vi "Read Parameters to process.vi"(8 "error in":errorcluster, 11 "Temperature Controller Logic runtime in":refnum<class "Temperature Controller Logic runtime.lvclass">) -> (0 "error out":errorcluster, 2 "Parameters to process":T1, 3 "Temperature Controller Logic runtime out":refnum<class "Temperature Controller Logic runtime.lvclass">)   [LabVIEW 2015, in "Temperature Controller Logic runtime.lvclass"]
uses:
  Temperature Controller Logic runtime.lvclass
  configuration/parameter data indices.ctl
  Temperature Controller Logic runtime.lvclass/Temperature Controller Logic runtime.ctl
  configuration/Temperature Controller Logic configuration.lvclass
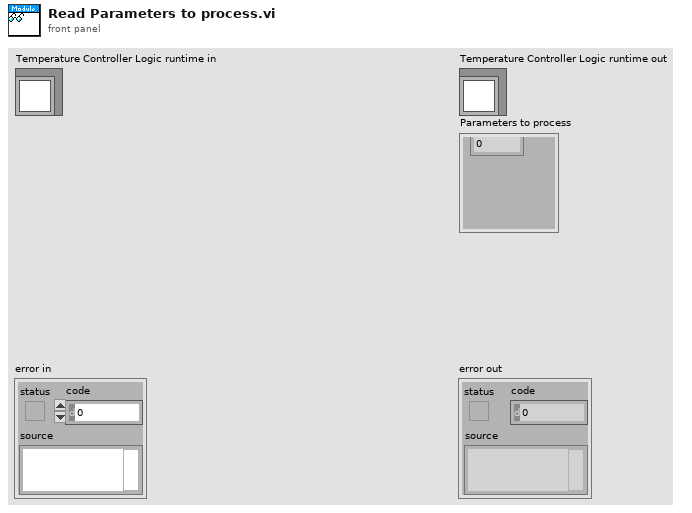
[diagram p1: front panel]
types:
  T1 = typedef "Temperature Controller Logic configuration.lvclass/parameter data indices.ctl" = cluster{"Double.Temperature":i32, "Double.setpoint":i32, "Double.output range high":i32, "Double.output range low":i32, "Double.Kc":i32, "Double.Ti":i32, "Double.Td":i32, "Boolean.Fan on?":i32}
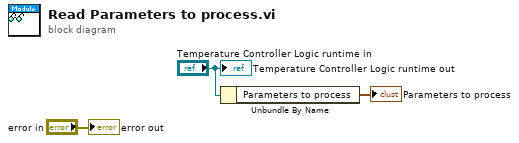
[diagram p0: block diagram]
diagram:
  n1 = Unbundle By Name("Temperature Controller Logic runtime in") -> ("Parameters to process"=→"Parameters to process":T1)
  "error out" <- "error in"
  "Temperature Controller Logic runtime out" <- "Temperature Controller Logic runtime in"
